vi "MoveColorArm.vi"(8 "Arm Valve State":T2, 11 "SecondaryJoystickButtons":T1) -> ()   [LabVIEW 2019]
uses:
  <vilib>/Rock Robotics/WPI/Solenoid/WPI_SolenoidValue.ctl
  Controls/SecondaryJoystickButtons.ctl
  <vilib>/Rock Robotics/WPI/Solenoid/WPI_SolenoidSetEnum.vi
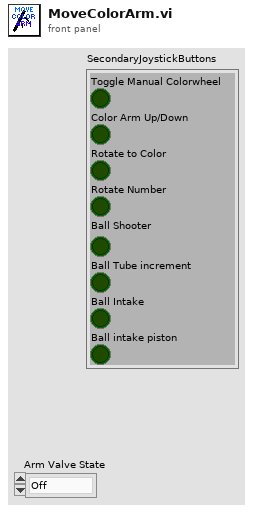
[diagram p1: front panel]
types:
  T1 = typedef "SecondaryJoystickButtons.ctl" = cluster{"Toggle Manual Colorwheel":bool, "Color Arm Up/Down":bool, "Rotate to Color":bool, "Rotate Number":bool, "Ball Shooter":bool, "Ball Tube increment":bool, "Ball Intake":bool, "Ball intake piston":bool}
  T2 = typedef "WPI_SolenoidValue.ctl" = enum16{"Off", "On", "Forward", "Reverse"}
  T3 = typedef "WPI_SolenoidDevRef.ctl" = cluster{"DevStatus":errorcluster, "Pneumatics Control Module":u8, "Forward Solenoid Channel":T4, "Reverse Solenoid Channel":T4}
  T4 = typedef "WPI_SolenoidChannel.ctl" = enum8{"Solenoid 0", "Solenoid 1", "Solenoid 2", "Solenoid 3", "Solenoid 4", "Solenoid 5", "Solenoid 6", "Solenoid 7", "Invalid"}
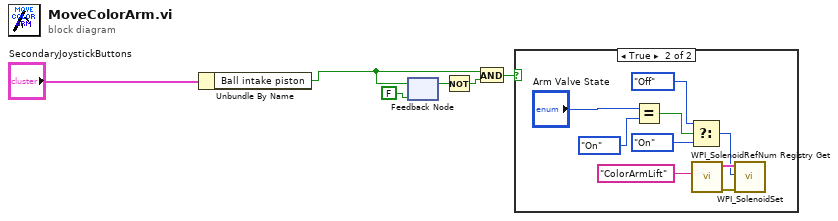
[diagram p0: block diagram]
diagram:
  n1 = Unbundle By Name("SecondaryJoystickButtons") -> ("Ball intake piston"=w1:bool)
  n2 = feedback-in #1(w1) -> ()
  n3 = feedback #1(FALSE ("Extend and Retract Arm")) -> (w5:bool)
  n4 = Not(x=w5) -> (.not. x?=w4:bool)
  n5 = And(x=w1, y=w4) -> (x .and. y?=w3:bool)
  n6 = case shown="True" w3 {
    frame False {
    }
    frame True {
      n7 = Equal?(x="Arm Valve State", y=WPI_SolenoidValue."On" ("Value")) -> (x = y?=w12:bool)
      n8 = Select(t=WPI_SolenoidValue."Off" ("Value"), s=w12, f=WPI_SolenoidValue."On" ("Value")) -> (s? t:f=w9:T2)
      n9 = call <vilib>:"WPI_SolenoidRefNum Registry Get.vi"("refnum name"="ColorArmLift") -> ("error out"=w14:errorcluster, "SolenoidDevRef"=w13:T3)  [unwired: 9 in]
      n10 = call-poly <vilib>:"WPI_SolenoidSet.vi"("error in (no error)"=w14, "Value"=w9, "SolenoidDevRef"=w13) -> ()  [unwired: 7 in, 2 out]
    }
  }
